vi "Convert State Value to Integer.vi"(11 "Floating Point State Value":dbl) -> (2 "Valid State Value":bool, 3 "Integer State Value":i32)   [LabVIEW 2020, in "Routing and Faulting Shared.lvlib"]
uses:
  Routing and Faulting Shared.lvlib
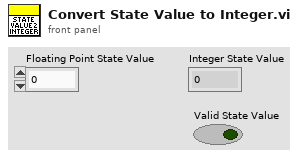
[diagram p1: front panel]
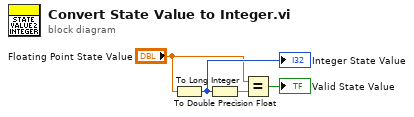
[diagram p0: block diagram]
diagram:
  n1 = To Long Integer(number="Floating Point State Value") -> (32bit integer=w3:i32)
  "Integer State Value" <- w3
  n2 = To Double Precision Float(number=w3) -> (double precision float=w2:dbl)
  n3 = Equal?(x="Floating Point State Value", y=w2) -> (x = y?=→"Valid State Value":bool)
